vi "GetAllBooks.vi"(1 "Author":string, 2 "directory":string) -> (0 "books":string[][](array[string]))   [LabVIEW 2012]
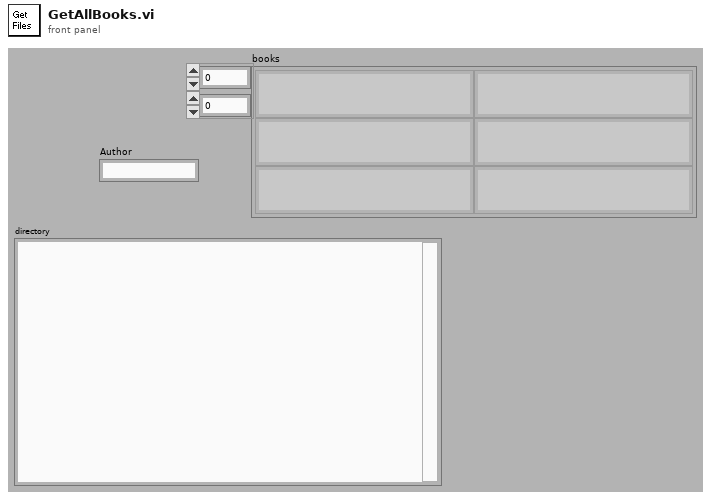
[diagram p1: front panel]
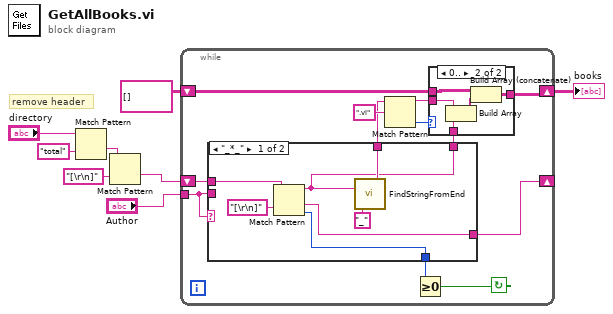
[diagram p0: block diagram]
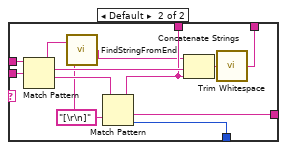
[diagram p2: hidden frame]
diagram:
  # "remove header"
  n1 = Match Pattern(string="directory", regular expression="total") -> (after substring=w3:string)  [unwired: 4 out]
  n2 = Match Pattern(string=w3, regular expression="[\r\n]") -> (after substring=w1:string)  [unwired: 4 out]
  n3 = while {
    shift-right: [w20] -> _
    shift-left: w1 -> [w11]
    tunnel: "Author" -> [w10]
    shift-right: [w14] -> w8
    shift-left: string[][] [] -> [w13]
    stop <- w18 continue-if-true
    n4 = case shown="\"_*_\"" w10 {
      tunnel: [w24 w38] -> w20
      tunnel: [w25 w37] -> w19
      tunnel: [w22 w33] -> w12
      tunnel: w10 -> [_ w36]
      tunnel: w11 -> [w26 w35]
      tunnel: [w21 w31] -> w9
      frame "_*_" {
        n5 = Match Pattern(string=w26, regular expression="[\r\n]") -> (before substring=w21:string, after substring=w24:string, offset past match=w25:i32)  [unwired: 2 out]
        n6 = call <userlib>:"FindStringFromEnd.vi"("regular expression"="_", "Full String"=w21) -> ("Remaining String"=w22:string)
      }
      frame Default {
        w29 = "[\r\n]" ("regular expression")
        n7 = Match Pattern(string=w35, regular expression=w36) -> (before substring=w30:string, match substring=w34:string, after substring=w39:string)  [unwired: 2 out]
        n8 = call <userlib>:"FindStringFromEnd.vi"("regular expression"=w29, "Full String"=w30) -> ("Remaining String"=w28:string)
        n9 = Match Pattern(string=w39, regular expression=w29) -> (before substring=w33:string, after substring=w38:string, offset past match=w37:i32)  [unwired: 2 out]
        n10 = Concatenate Strings(w28, w34, w33) -> (w32:string)
        n11 = call <vilib>:"Trim Whitespace.vi"("string"=w32) -> ("trimmed string"=w31:string)  [unwired: 1 in]
      }
    }
    n12 = Match Pattern(string=w12, regular expression=".vi") -> (before substring=w15:string, offset past match=w16:i32)  [unwired: 3 out]
    n13 = Greater Or Equal To 0?(x=w19) -> (x >= 0?=w18:bool)
    n14 = case shown="0.." w16 {
      tunnel: w15 -> [_ w43]
      tunnel: [w40 w45] -> w14
      tunnel: w13 -> [w40 w44]
      tunnel: w9 -> [_ w42]
      frame ..-1 {
      }
      frame 0.. {
        n15 = Build Array(w43, w42) -> (w41:string[])
        n16 = Build Array (concatenate)(w44, w41) -> (w45:string[][])
      }
    }
  }
  "books" <- w8
